vi "Build.vi"(8 "error in (no error)":errorcluster, 9 "build":bool, 11 "Class in":refnum<class "AB_UI_Frmwk_Installer.lvclass">) -> (0 "error out":errorcluster, 3 "Class out":refnum<class "AB_UI_Frmwk_Installer.lvclass">)   [LabVIEW 2020, in "AB_UI_Frmwk_Installer.lvclass"]
uses:
  <vilib>/AppBuilder/IB_Classes/Installer/UI/AB_UI_Frmwk_Installer.lvclass
  <vilib>/AppBuilder/IB_Classes/Installer/UI/AB_UI_Frmwk_Installer.lvclass/AB_UI_Frmwk_Installer.ctl
  <resource>/Framework/Providers/Builds/Installer/SRdB/IB_SRdB_Action.ctl
  <resource>/Framework/Providers/Builds/Installer/SRdb_Bld/SRdB_Bld_action.ctl
  <resource>/Framework/Providers/Builds/Installer/SRdB_Proj/SRdB_Proj_Action.ctl
  <resource>/Framework/Providers/Builds/Installer/SRdB_Icon/SRdB_Icon_action.ctl
  <vilib>/AppBuilder/IB_Classes/Installer/Installer.lvclass
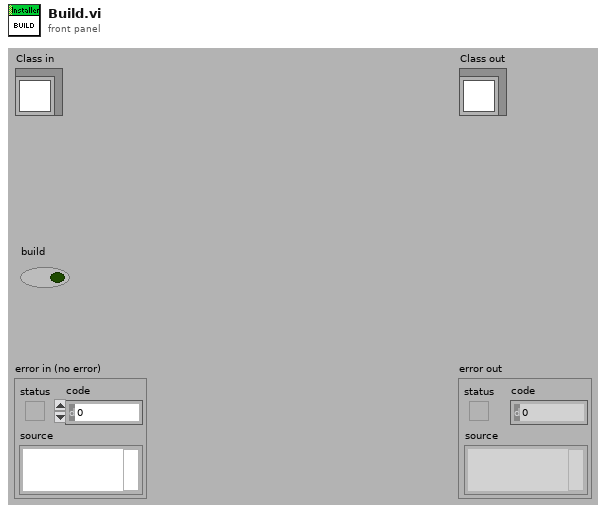
[diagram p1: front panel]
types:
  T1 = typedef "SRdB_Icon_action.ctl" = enum16{"read", "write", "create", "delete", "initialize", "unInitialize", "getLock", "readAll", "writeAll"}
  T2 = typedef "SRdB_Proj_Action.ctl" = enum16{"read", "write", "create", "delete", "initialize", "unInitialize", "getLock", "readAll", "writeAll"}
  T3 = typedef "SRdB_Bld_action.ctl" = enum16{"read", "write", "create", "delete", "initialize", "unInitialize", "getLock", "readAll", "writeAll"}
  T4 = typedef "IB_SRdB_Action.ctl" = enum16{"read", "write", "create", "delete", "initialize", "unInitialize", "getLock", "readAll", "writeAll"}
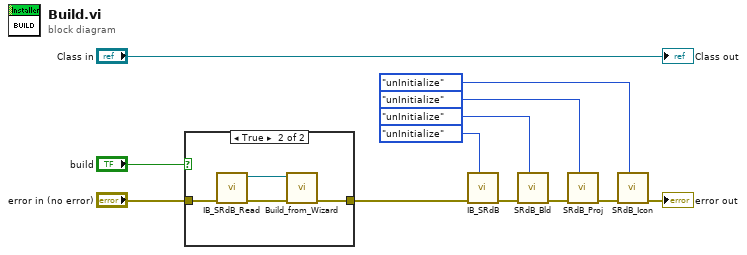
[diagram p0: block diagram]
diagram:
  n1 = case shown="True" "build" {
    tunnel: "error in (no error)" -> [w13 w17]
    tunnel: [w13 w16] -> w11
    frame False {
    }
    frame True {
      n2 = call <resource>:"IB_SRdB_Read.vi"("error in (no error)"=w17) -> ("error out"=w14:errorcluster, "installer out"=w15:refnum<class "Installer.lvclass">)  [unwired: 9 in]
      n3 = call-dynamic "Build_from_Wizard.vi"("error in (no error)"=w14, "Class in"=w15) -> ("error out"=w16:errorcluster)  [unwired: 8 in, 1 out]
    }
  }
  n4 = call <resource>:"IB_SRdB.vi"("action"=IB_SRdB_Action."unInitialize", "error in (no error)"=w11) -> ("error out"=w7:errorcluster)  [unwired: 7 in, 2 out]
  n5 = call <resource>:"SRdB_Bld.vi"("action"=SRdB_Bld_action."unInitialize", "error in (no error)"=w7) -> ("error out"=w4:errorcluster)  [unwired: 7 in, 2 out]
  n6 = call <resource>:"SRdB_Proj.vi"("action"=SRdB_Proj_Action."unInitialize", "error in (no error)"=w4) -> ("error out"=w5:errorcluster)  [unwired: 7 in, 2 out]
  n7 = call <resource>:"SRdB_Icon.vi"("action"=SRdB_Icon_action."unInitialize", "error in (no error)"=w5) -> ("error out"=→"error out":errorcluster)  [unwired: 7 in, 2 out]
  "Class out" <- "Class in"
